vi "Preallocate Method Results.vi"(9 "Test Methods":string[](array[string]), 10 "Test Case":string, 11 "Test Case Result in":refnum<class "Test Case Result.lvclass">) -> (3 "Test Case Result out":refnum<class "Test Case Result.lvclass">)   [LabVIEW 2020, in "Test Case Result.lvclass"]
uses:
  Test Case Result.lvclass
  Method Result/Method Result.lvclass
  Method Result/Method Result.lvclass/Method Result.ctl
  Test Case Result.lvclass/Test Case Result.ctl
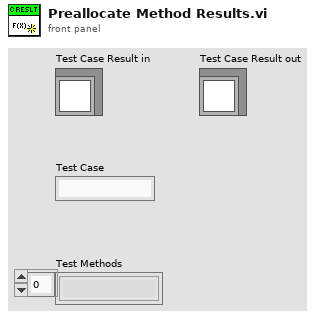
[diagram p1: front panel]
types:
  T1 = map{string, refnum<class "Method Result.lvclass">}
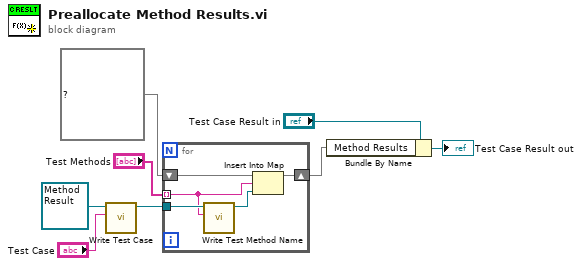
[diagram p0: block diagram]
diagram:
  n1 = call "Write Test Case.vi"("Test Case"="Test Case", "Method Result In"=refnum<class "Method Result.lvclass"> refnum ("value")) -> ("Method Result Out"=w5:refnum<class "Method Result.lvclass">)  [unwired: 9 in]
  n2 = for {
    shift-right: [w12] -> w1
    shift-left: T1 {} ("Method Results") -> [w13]
    tunnel: w5 -> [w11]
    tunnel: "Test Methods" -> [w9] mode=indexing
    n3 = call "Write Test Method Name.vi"("Test Method Name"=w9, "Method Result In"=w11) -> ("Method Result Out"=w10:refnum<class "Method Result.lvclass">)  [unwired: 9 in]
    n4 = Insert Into Map(map in=w13, key=w9, value=w10) -> (map out=w12:T1)  [unwired: 2 out]
  }
  n5 = Bundle By Name(cluster="Test Case Result in", "Method Results"=w1) -> (→"Test Case Result out":refnum<class "Test Case Result.lvclass">)
